vi "Add Information Channels.vi"(8 "error in (no error)":errorcluster, 11 "Node Ptr":u64) -> (0 "error out":errorcluster, 3 "Parent Ref out":T1 format="%.0x")   [LabVIEW 2023, in "J1939 Addon Shared.lvlib"]
uses:
  J1939 Addon Shared.lvlib
  <vilib>/NI VeriStand/Custom Device API/Custom Device Item Ref.ctl
  <vilib>/NI VeriStand/Custom Device API/Custom Device Channel.ctl
  <vilib>/NI VeriStand/Custom Device API/Custom Device Channel Type.ctl
  Constants.vi
  <vilib>/NI VeriStand/Custom Device API/Custom Device API.lvlib
  <vilib>/NI/NI VeriStand Advanced SysDef API/SysDef API/Advanced System Definition.lvlib
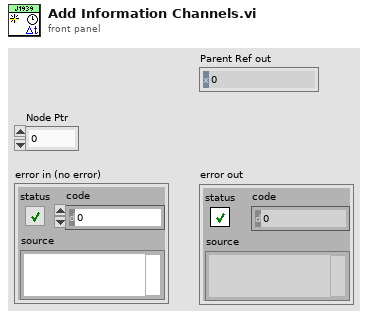
[diagram p1: front panel]
types:
  T1 = typedef "Custom Device API.lvlib/Custom Device Item Ref.ctl" = u64
  T2 = typedef "Custom Device API.lvlib/Custom Device Channel.ctl" = cluster{"Type":T3, "Units":string, "Default Value":dbl, "Faultable":bool, "Scalable":bool}
  T3 = typedef "Custom Device API.lvlib/Custom Device Channel Type.ctl" = enum16{"Input", "Output"}
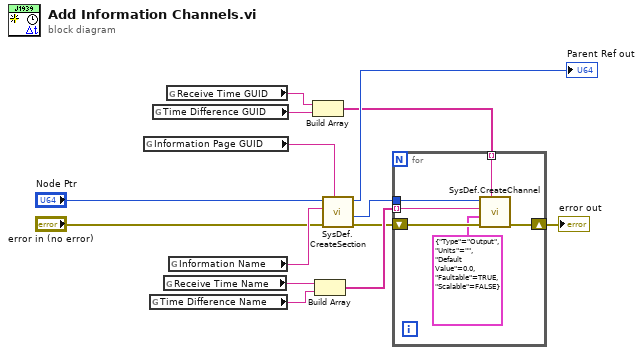
[diagram p0: block diagram]
diagram:
  n1 = global read "Constants.vi" "Information Page GUID"() -> (w6:string)
  n2 = global read "Constants.vi" "Time Difference Name"() -> (w9:string)
  n3 = global read "Constants.vi" "Time Difference GUID"() -> (w11:string)
  n4 = global read "Constants.vi" "Receive Time Name"() -> (w8:string)
  n5 = global read "Constants.vi" "Receive Time GUID"() -> (w12:string)
  n6 = global read "Constants.vi" "Information Name"() -> (w7:string)
  n7 = Build Array(w12, w11) -> (w13:string[])
  n8 = Build Array(w8, w9) -> (w10:string[])
  n9 = call <vilib>:"SysDef.CreateSection.vi"("GUID"=w6, "error in (no error)"="error in (no error)", "Name"=w7, "nodeID"="Node Ptr") -> ("error out"=w2:errorcluster, "New NodeID"=w3:u64, "nodeID out"=→"Parent Ref out":u64)  [unwired: 4 in, 1 out]
  n10 = for {
    tunnel: w3 -> [w19]
    shift-right: [w18] -> w5
    shift-left: w2 -> [w20]
    tunnel: w13 -> [w16] mode=indexing
    tunnel: w10 -> [w15] mode=indexing
    n11 = call <vilib>:"SysDef.CreateChannel.vi"("GUID"=w16, "error in (no error)"=w20, "Channel"=T2 {"Type"=enum."Output", "Units"="", "Default Value"=0.0, "Faultable"=TRUE, "Scalable"=FALSE}, "Name"=w15, "nodeID"=w19) -> ("error out"=w18:errorcluster)  [unwired: 3 in, 3 out]
  }
  "error out" <- w5
